vi "Quadratic Roots.vi"() -> ()   [LabVIEW 2021]
uses:
  <vilib>/express/express arith-compare/Formula/XNode/ExpressFormulaBlockNode.xnode
panel:
  out "Quadratic Plot":cluster{"X":dbl, "Y":dbl}[](graph)
  out "Root 2":dbl
  out "Root 1":dbl
  in  "C":dbl
  in  "B":dbl
  in  "A":dbl
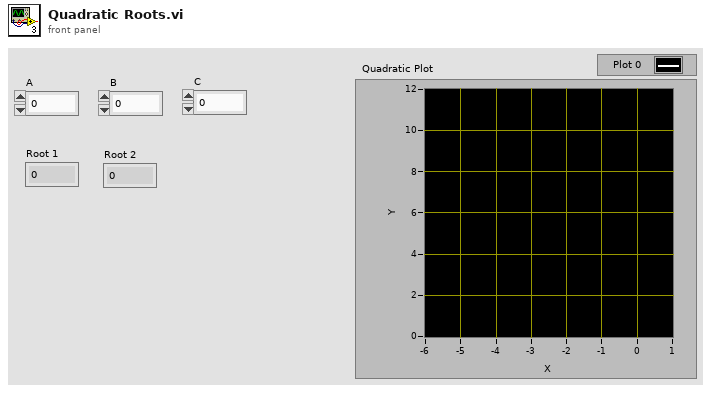
[diagram p1: front panel]
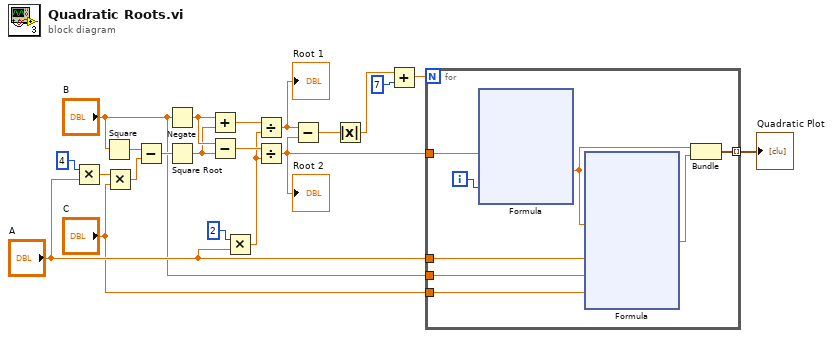
[diagram p0: block diagram]
diagram:
  n1 = Multiply(x=4, y="A") -> (x*y=w20:dbl)
  n2 = Square(x="B") -> (x^2=w19:dbl)
  n3 = Multiply(x=w20, y="C") -> (x*y=w18:dbl)
  n4 = Subtract(x=w19, y=w18) -> (x-y=w17:dbl)
  n5 = Negate(x="B") -> (-x=w16:dbl)
  n6 = Square Root(x=w17) -> (sqrt(x)=w15:dbl)
  n7 = Add(x=w16, y=w15) -> (x+y=w14:dbl)
  n8 = Subtract(x=w16, y=w15) -> (x-y=w13:dbl)
  n9 = Multiply(x=2, y="A") -> (x*y=w11:dbl)
  n10 = Divide(x=w14, y=w11) -> (x/y=w10:dbl)
  "Root 1" <- w10
  n11 = Divide(x=w13, y=w11) -> (x/y=w2:dbl)
  "Root 2" <- w2
  n12 = Subtract(x=w10, y=w2) -> (x-y=w9:dbl)
  n13 = Absolute Value(x=w9) -> (abs(x)=w8:dbl)
  n14 = Add(x=w8, y=7) -> (x+y=w6:dbl)
  n15 = for {
    N: w6 -> [_]
    tunnel: "A" -> [w29]
    tunnel: "B" -> [w28]
    tunnel: "C" -> [w27]
    tunnel: w2 -> [w26]
    tunnel: [w22] -> w1 mode=indexing
    i -> [w25]
    n16 = xnode "Formula"("R2"=w26, "I"=w25) -> ("Result"=w24:dbl)  [unwired: 1 in, 1 out]
    n17 = xnode "Formula"("X"=w24, "A"=w29, "B"=w28, "C"=w27) -> ("Result"=w23:dbl)  [unwired: 1 in, 1 out]
    n18 = Bundle("Result"=w24, "Result"=w23) -> (w22:cluster{"Result":dbl, "Result":dbl})  [unwired: 1 in]
  }
  "Quadratic Plot" <- w1
